vi "SRV_PM_Data Byte Stuffing.vi"(0 "Data":u8[](array[numeric]) format="%.0x", 11 "error in (no error)":errorcluster) -> (4 "Data dup":u8[](array[numeric]) format="%.0x", 8 "Stuffed Data":u8[](array[numeric]) format="%.0x", 15 "error out":errorcluster)   [LabVIEW 2014]
panel:
  in  "Stuffing Byte (0x00)":u8 format="%.0x"
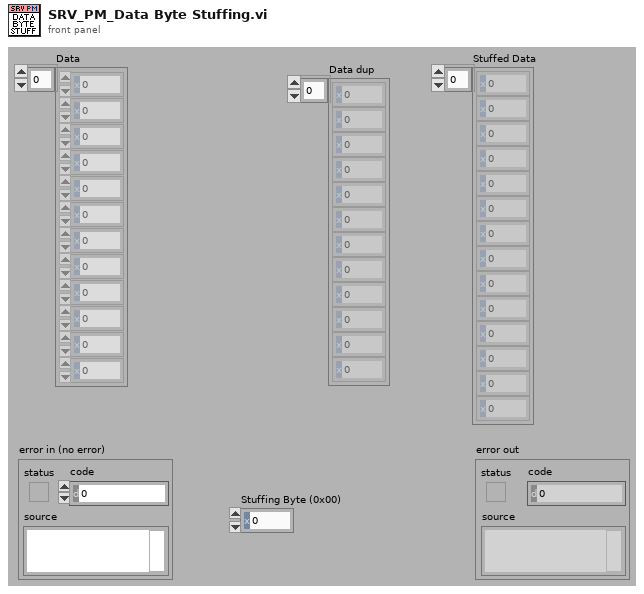
[diagram p1: front panel]
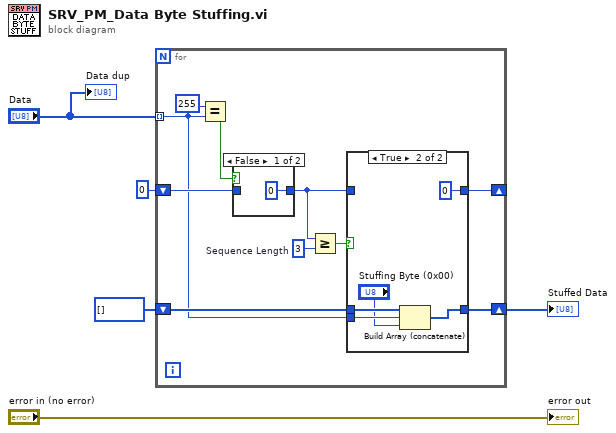
[diagram p0: block diagram]
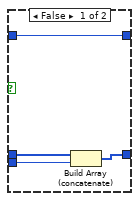
[diagram p2: hidden frame]
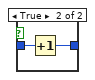
[diagram p3: hidden frame]
diagram:
  n1 = for {
    tunnel: "Data" -> [w6] mode=indexing
    shift-right: [w10] -> _
    shift-left: 0 -> [w13]
    shift-right: [w7] -> w3
    shift-left: u8[] [] ("Stuffed Data") -> [w8]
    w12 = 3  # Sequence Length
    n2 = Equal?(x=u8 255, y=w6) -> (x = y?=w14:bool)
    n3 = case shown="False" w14 {
      tunnel: w13 -> [_ w27]
      tunnel: [0 w26] -> w11
      frame False {
      }
      frame True {
        n4 = Increment(x=w27) -> (x+1=w26:i32)
      }
    }
    n5 = Greater Or Equal?(x=w11, y=w12) -> (x >= y?=w9:bool)
    n6 = case shown="True" w9 {
      tunnel: w11 -> [w19 _]
      tunnel: [w19 0] -> w10
      tunnel: w8 -> [w17 w22]
      tunnel: [w18 w23] -> w7
      tunnel: w6 -> [w16 w21]
      frame False {
        n7 = Build Array (concatenate)(w17, w16) -> (w18:u8[])
      }
      frame True {
        n8 = Build Array (concatenate)(w22, w21, "Stuffing Byte (0x00)") -> (w23:u8[])
      }
    }
  }
  "Stuffed Data" <- w3
  "error out" <- "error in (no error)"
  "Data dup" <- "Data"
